vi "循环扫描脚本.vi"(6 "4-wire":bool, 8 "扫描":T1 {"测试参数"."反向极限电流(mA)" min=0.0 max=3000.0; "测试参数"."反向电压(V)" min=-40.0 max=40.0; "测试参数"."正向极限电流(mA)" min=0.0 max=3000.0; "测试参数"."正向电压(V)" min=-40.0 max=40.0; "时序参数"."反改变量(V)" min=0.0 max=40.0 step=5e-06; "时序参数"."正改变量(V)" min=0.0 max=40.0 step=5e-06; "时序参数"."nplc" min=0.001}, 10 "错误输入（无错误）":errorcluster) -> (2 "错误输出":errorcluster, 3 "Script":string)   [LabVIEW 2020]
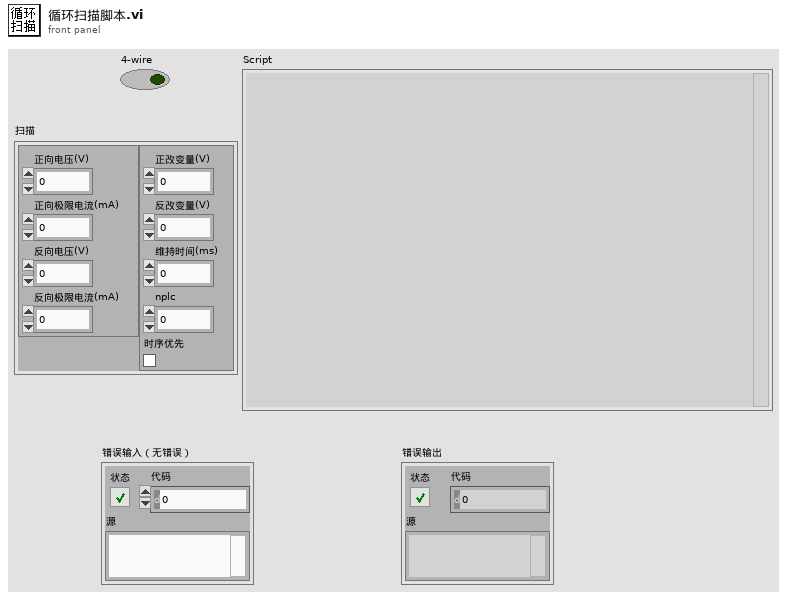
[diagram p1: front panel]
types:
  T1 = typedef "扫描参数.ctl" = cluster{"测试参数":cluster{"正向电压(V)":dbl, "正向极限电流(mA)":dbl, "反向电压(V)":dbl, "反向极限电流(mA)":dbl}, "时序参数":cluster{"正改变量(V)":dbl, "反改变量(V)":dbl, "维持时间(ms)":dbl, "nplc":dbl, "时序优先":bool}}
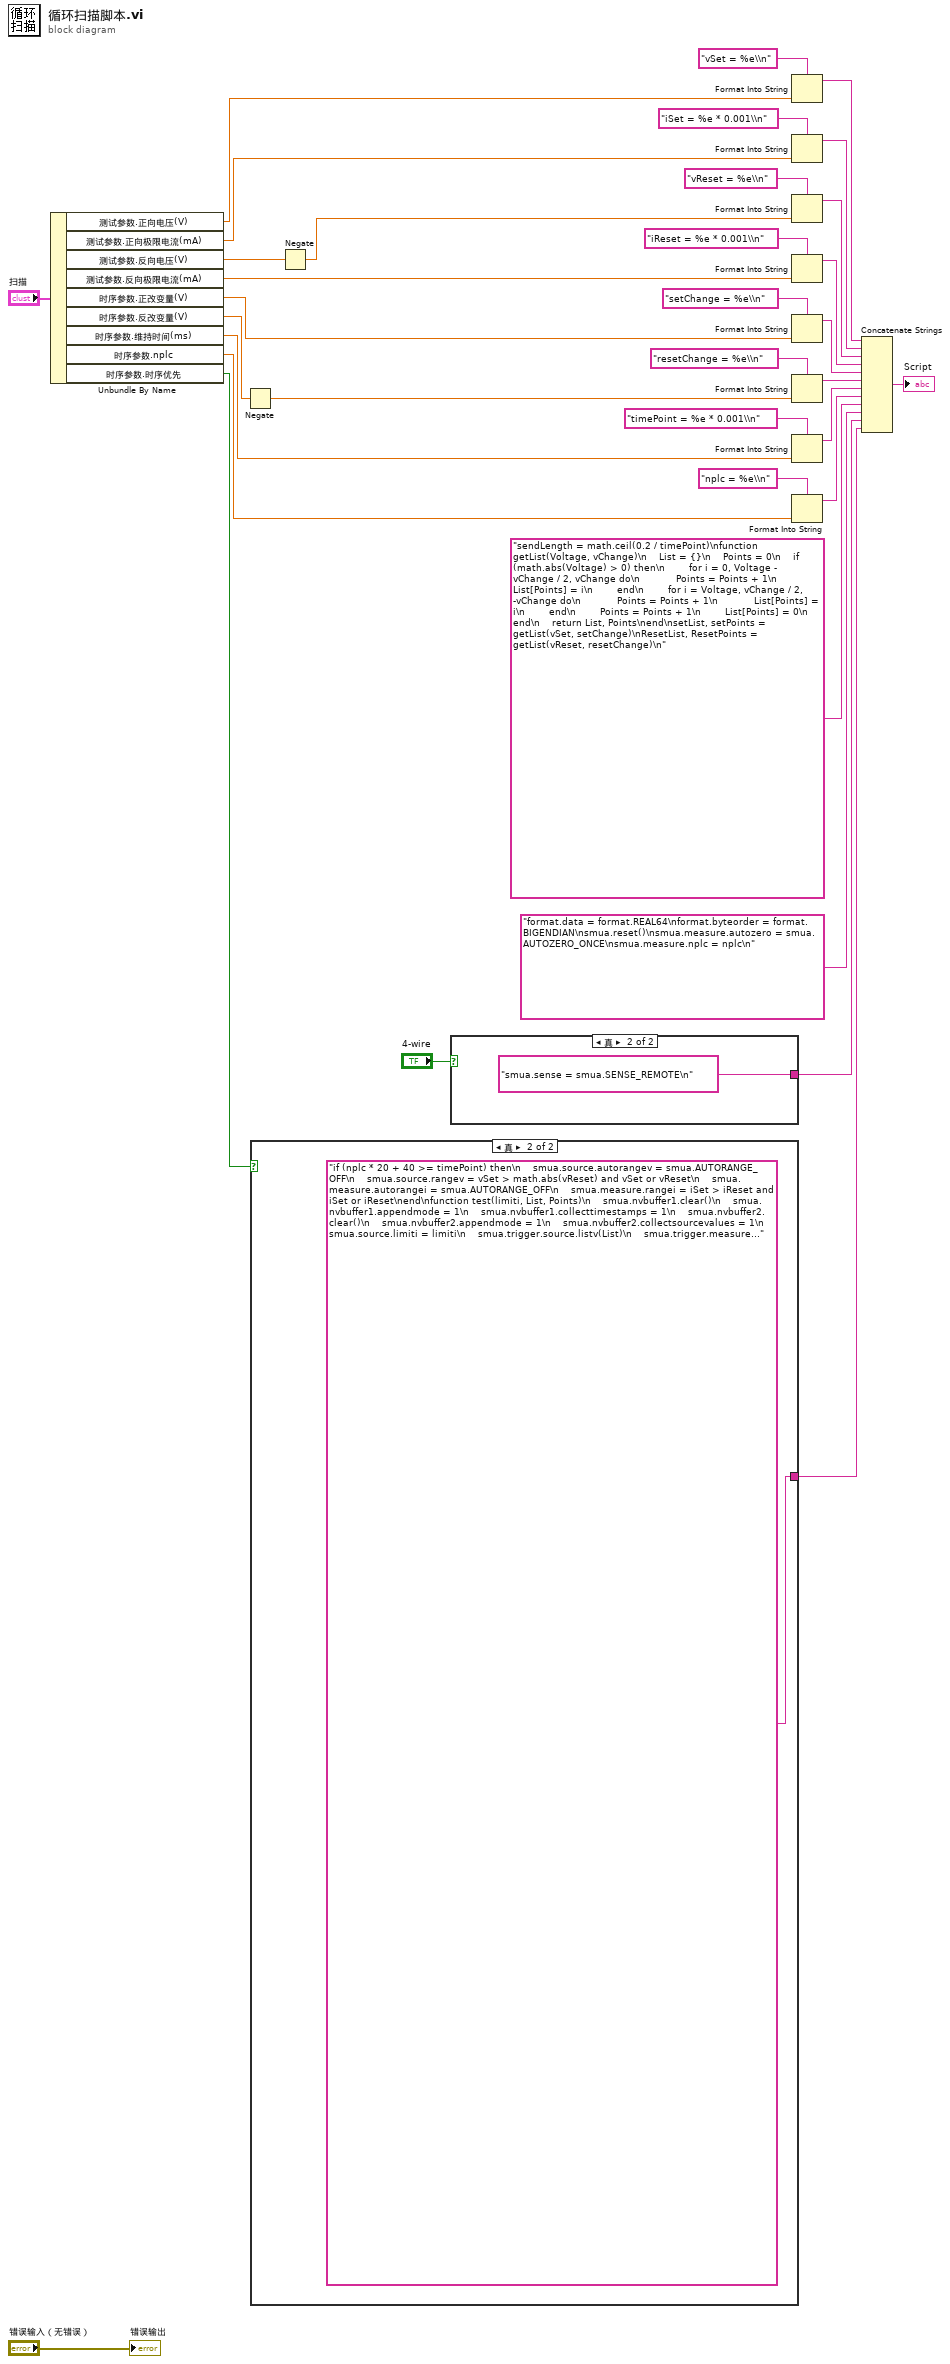
[diagram p0: block diagram]
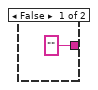
[diagram p2: hidden frame]
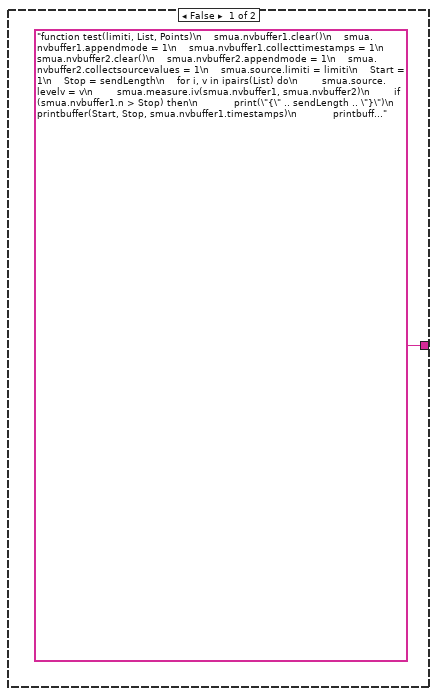
[diagram p3: hidden frame]
diagram:
  n1 = Unbundle By Name("扫描") -> ("测试参数.正向电压(V)"=w12:dbl, "测试参数.正向极限电流(mA)"=w11:dbl, "测试参数.反向电压(V)"=w10:dbl, "测试参数.反向极限电流(mA)"=w9:dbl, "时序参数.正改变量(V)"=w8:dbl, "时序参数.反改变量(V)"=w3:dbl, "时序参数.维持时间(ms)"=w17:dbl, "时序参数.nplc"=w18:dbl, "时序参数.时序优先"=w6:bool)
  n2 = Negate(x=w3) -> (-x=w1:dbl)
  n3 = case shown="真" w6 {
    tunnel: ["function test(limiti, List, Points)\n    smua.nvbuffer1.clear()\n    smua.nvbuffer1.appendmode = 1\n    smua.nvbuffer1.collecttimestamps = 1\n    smua.nvbuffer2.clear()\n    smua.nvbuffer2.appendmode = 1\n    smua.nvbuffer2.collectsourcevalues = 1\n    smua.source.limiti = limiti\n    Start = 1\n    Stop = sendLength\n    for i, v in ipairs(List) do\n        smua.source.levelv = v\n        smua.measure.iv(smua.nvbuffer1, smua.nvbuffer2)\n        if (smua.nvbuffer1.n > Stop) then\n            print(\"{\" .. sendLength .. \"}\")\n            printbuffer(Start, Stop, smua.nvbuffer1.timestamps)\n            printbuffer(Start, Stop, smua.nvbuffer2.sourcevalues)\n            printbuffer(Start, Stop, smua.nvbuffer1)\n            printbuffer(Start, Stop, smua.nvbuffer2)\n            Start = Start + sendLength\n            Stop = Stop + sendLength\n        end\n    end\n    Stop = Points\n    print(\"{\" .. Stop - Start + 1 .. \"}\")\n    printbuffer(Start, Stop, smua.nvbuffer1.timestamps)\n    printbuffer(Start, Stop, smua.nvbuffer2.sourcevalues)\n    printbuffer(Start, Stop, smua.nvbuffer1)\n    printbuffer(Start, Stop, smua.nvbuffer2)\n    print(\"{done}\")\nend\nsmua.source.output = smua.OUTPUT_ON\nif (setPoints > 0) then test(iSet, setList, setPoints) end\nif (ResetPoints > 0) then test(iReset, ResetList, ResetPoints) end\nsmua.source.output = smua.OUTPUT_OFF\nreset()\n" "if (nplc * 20 + 40 >= timePoint) then\n    smua.source.autorangev = smua.AUTORANGE_OFF\n    smua.source.rangev = vSet > math.abs(vReset) and vSet or vReset\n    smua.measure.autorangei = smua.AUTORANGE_OFF\n    smua.measure.rangei = iSet > iReset and iSet or iReset\nend\nfunction test(limiti, List, Points)\n    smua.nvbuffer1.clear()\n    smua.nvbuffer1.appendmode = 1\n    smua.nvbuffer1.collecttimestamps = 1\n    smua.nvbuffer2.clear()\n    smua.nvbuffer2.appendmode = 1\n    smua.nvbuffer2.collectsourcevalues = 1\n    smua.source.limiti = limiti\n    smua.trigger.source.listv(List)\n    smua.trigger.measure.iv(smua.nvbuffer1, smua.nvbuffer2)\n    smua.trigger.source.stimulus = trigger.timer[1].EVENT_ID\n    smua.trigger.source.action = smua.ENABLE\n    smua.trigger.measure.action = smua.ENABLE\n    smua.trigger.count = Points\n    smua.trigger.arm.stimulus = trigger.EVENT_ID\n    trigger.timer[1].reset()\n    trigger.timer[1].stimulus = smua.trigger.ARMED_EVENT_ID\n    trigger.timer[1].passthrough = false\n    trigger.timer[1].delay = timePoint\n    trigger.timer[1].count = Points\n    smua.trigger.initiate()\n    smua.trigger.arm.set()\nend\nfunction sendData()\n    Start = 1\n    Stop = sendLength\n    repeat\n        if (bit.test(status.operation.instrument.smua.condition, 4) == false) then\n            break\n        elseif (smua.nvbuffer1.n > Stop) then\n            print(\"{\" .. sendLength .. \"}\")\n            printbuffer(Start, Stop, smua.nvbuffer1.timestamps)\n            printbuffer(Start, Stop, smua.nvbuffer2.sourcevalues)\n            printbuffer(Start, Stop, smua.nvbuffer1)\n            printbuffer(Start, Stop, smua.nvbuffer2)\n            Start = Start + sendLength\n            Stop = Stop + sendLength\n        end\n        delay(timePoint)\n    until (false)\n    Stop = smua.nvbuffer1.n\n    print(\"{\" .. Stop - Start + 1 .. \"}\")\n    printbuffer(Start, Stop, smua.nvbuffer1.timestamps)\n    printbuffer(Start, Stop, smua.nvbuffer2.sourcevalues)\n    printbuffer(Start, Stop, smua.nvbuffer1)\n    printbuffer(Start, Stop, smua.nvbuffer2)\n    print(\"{done}\")\nend\nsmua.source.output = smua.OUTPUT_ON\nif (setPoints > 0) then\n    test(iSet, setList, setPoints)\n    sendData()\nend\nif (ResetPoints > 0) then\n    test(iReset, ResetList, ResetPoints)\n    sendData()\nend\nsmua.source.output = smua.OUTPUT_OFF\nreset()\n"] -> w27
    frame False {
    }
    frame True {
    }
  }
  n4 = Negate(x=w10) -> (-x=w7:dbl)
  n5 = case shown="真" "4-wire" {
    tunnel: ["" "smua.sense = smua.SENSE_REMOTE\n"] -> w26
    frame False {
    }
    frame True {
    }
  }
  n6 = Format Into String(format string="vSet = %e\\n" ("格式字符串"), w12) -> (resulting string=w14:string)  [unwired: 2 in, 1 out]
  n7 = Format Into String(format string="iSet = %e * 0.001\\n" ("格式字符串"), w11) -> (resulting string=w13:string)  [unwired: 2 in, 1 out]
  n8 = Format Into String(format string="vReset = %e\\n" ("格式字符串"), w7) -> (resulting string=w32:string)  [unwired: 2 in, 1 out]
  n9 = Format Into String(format string="iReset = %e * 0.001\\n" ("格式字符串"), w9) -> (resulting string=w22:string)  [unwired: 2 in, 1 out]
  n10 = Format Into String(format string="setChange = %e\\n" ("格式字符串"), w8) -> (resulting string=w23:string)  [unwired: 2 in, 1 out]
  n11 = Format Into String(format string="resetChange = %e\\n" ("格式字符串"), w1) -> (resulting string=w2:string)  [unwired: 2 in, 1 out]
  n12 = Format Into String(format string="timePoint = %e * 0.001\\n", w17) -> (resulting string=w21:string)  [unwired: 2 in, 1 out]
  n13 = Format Into String(format string="nplc = %e\\n", w18) -> (resulting string=w20:string)  [unwired: 2 in, 1 out]
  n14 = Concatenate Strings(w14, w13, w32, w22, w23, w2, w21, w20, "sendLength = math.ceil(0.2 / timePoint)\nfunction getList(Voltage, vChange)\n    List = {}\n    Points = 0\n    if (math.abs(Voltage) > 0) then\n        for i = 0, Voltage - vChange / 2, vChange do\n            Points = Points + 1\n            List[Points] = i\n        end\n        for i = Voltage, vChange / 2, -vChange do\n            Points = Points + 1\n            List[Points] = i\n        end\n        Points = Points + 1\n        List[Points] = 0\n    end\n    return List, Points\nend\nsetList, setPoints = getList(vSet, setChange)\nResetList, ResetPoints = getList(vReset, resetChange)\n", "format.data = format.REAL64\nformat.byteorder = format.BIGENDIAN\nsmua.reset()\nsmua.measure.autozero = smua.AUTOZERO_ONCE\nsmua.measure.nplc = nplc\n", w26, w27) -> (→"Script":string)
  "错误输出" <- "错误输入（无错误）"
